vi "Write XY.vi"(9 "X":dbl[](array[numeric]), 10 "Y":dbl[](array[numeric]), 11 "Scale_PiecedLinear in":refnum<class "Scale_PiecedLinear.lvclass">) -> (3 "Scale_PiecedLinear out":refnum<class "Scale_PiecedLinear.lvclass">)   [LabVIEW 2019, in "Scale_PiecedLinear.lvclass"]
uses:
  Scale_PiecedLinear.lvclass
  Scale_PiecedLinear.lvclass/Scale_PiecedLinear.ctl
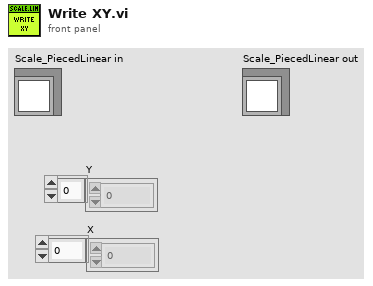
[diagram p1: front panel]
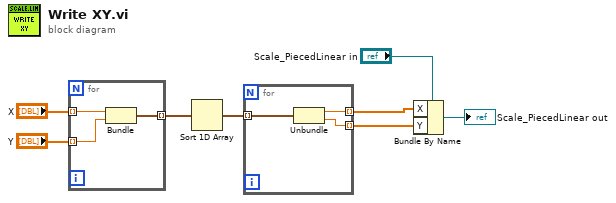
[diagram p0: block diagram]
diagram:
  n1 = for {
    tunnel: "X" -> [w11] mode=indexing
    tunnel: "Y" -> [w10] mode=indexing
    tunnel: [w9] -> w4 mode=indexing
    n2 = Bundle("X"=w11, "X"=w10) -> (w9:cluster{"X":dbl, "X":dbl})  [unwired: 1 in]
  }
  n3 = Sort 1D Array(array=w4) -> (sorted array=w3:cluster{"X":dbl, "X":dbl}[])
  n4 = for {
    tunnel: w3 -> [w14] mode=indexing
    tunnel: [w13] -> w2 mode=indexing
    tunnel: [w12] -> w1 mode=indexing
    n5 = Unbundle(w14) -> ("X"=w13:dbl, "X"=w12:dbl)
  }
  n6 = Bundle By Name(cluster="Scale_PiecedLinear in", "X"=w2, "Y"=w1) -> (→"Scale_PiecedLinear out":refnum<class "Scale_PiecedLinear.lvclass">)
